vi "Multimetr-facade.vi"(0 "Data In":T4, 2 "Display State In":T2 {"Mode" items=["U DC", "U AC", "I DC", "I AC", "R"]}, 3 "Container State":T3) -> (6 "Data Out":T4, 7 "Display State Out":T2 {"Mode" items=["U DC", "U AC", "I DC", "I AC", "R"]}, 8 "Action":T1)   [LabVIEW 2020, in "Multimetr.xctl"]
uses:
  Multimetr.xctl
  Multimetr-data.ctl
  <vilib>/_xctls/Container State.ctl
  Multimetr-state.ctl
  <vilib>/_xctls/Action.ctl
  <vilib>/_xctls/XControlSupport.lvlib
panel:
  out "U/I/R":dbl
  in  "Power":bool
  in  "Knob":u8(knob)=3 min=3 max=7 step=1 scale=0.0..10.0
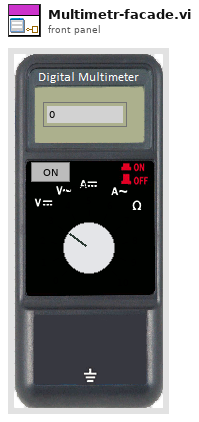
[diagram p1: front panel]
types:
  T1 = typedef "XControlSupport.lvlib/Action.ctl" = cluster{"Data Changed?":bool, "State Changed?":bool, "Action Name":string}
  T2 = typedef "Multimetr.xctl/Multimetr-state.ctl" = cluster{"ON":bool, "Mode":u16, "I connected?":bool, "U connected?":bool}
  T3 = typedef "XControlSupport.lvlib/Container State.ctl" = cluster{"Indicator?":bool, "Run Mode?":bool, " Refnum":refnum<vi>}
  T4 = typedef "Multimetr.xctl/Multimetr-data.ctl" = cluster{"Data":dbl, "Power":bool}
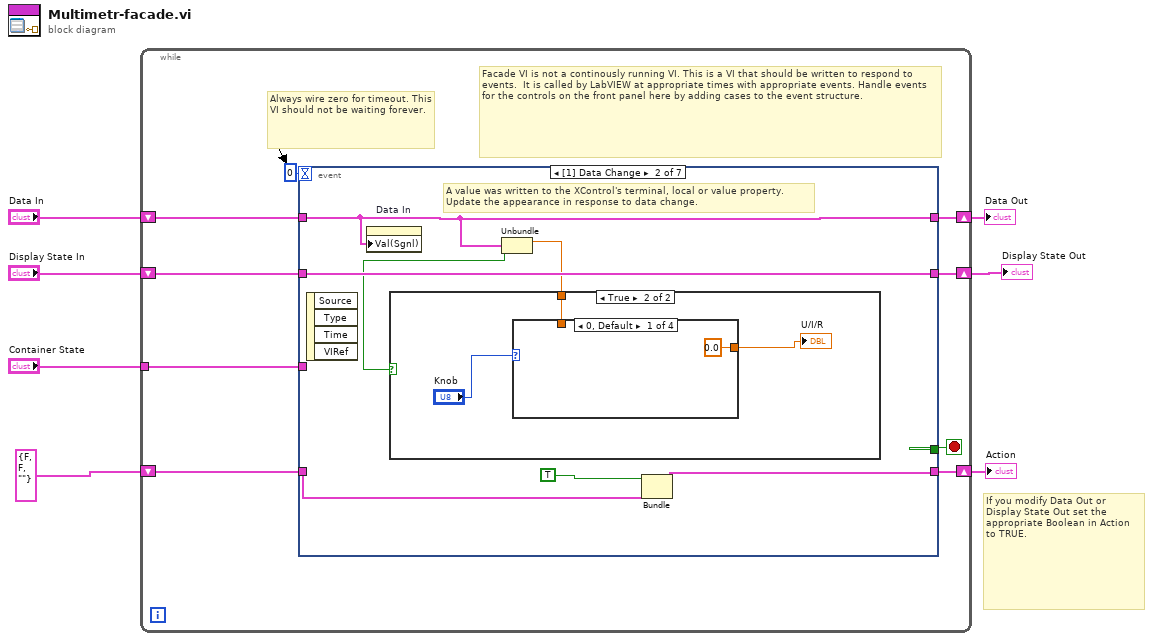
[diagram p0: block diagram]
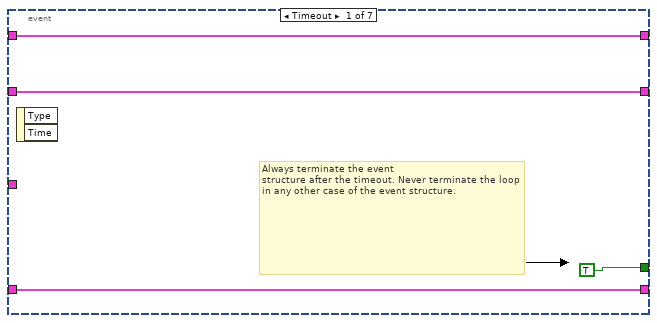
[diagram p2: hidden frame]
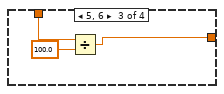
[diagram p5: hidden frame]
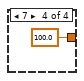
[diagram p6: hidden frame]
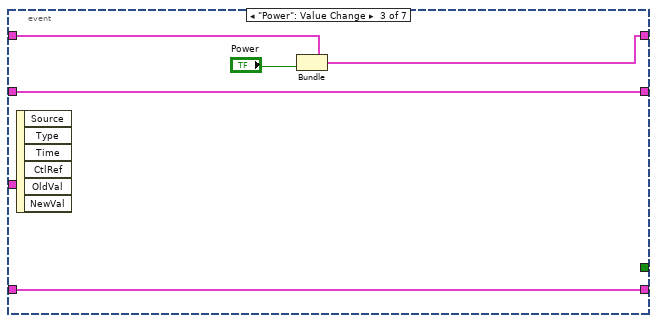
[diagram p7: hidden frame]
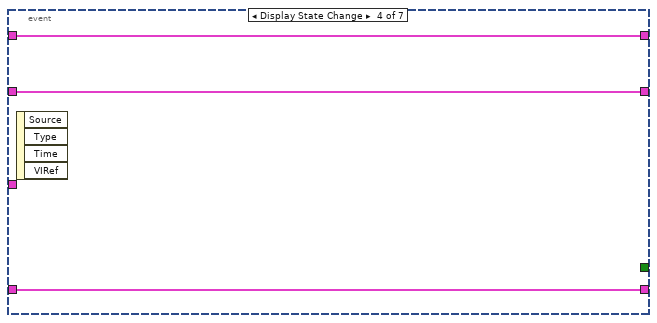
[diagram p8: hidden frame]
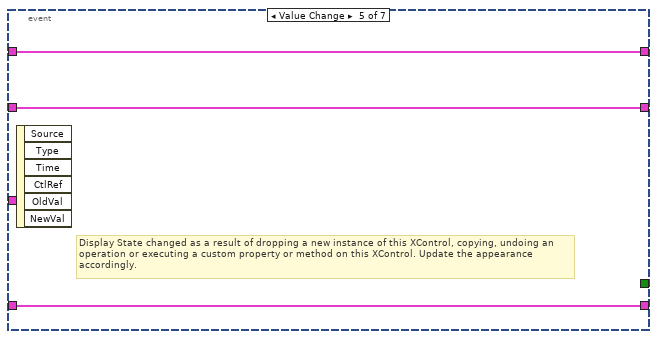
[diagram p9: hidden frame]
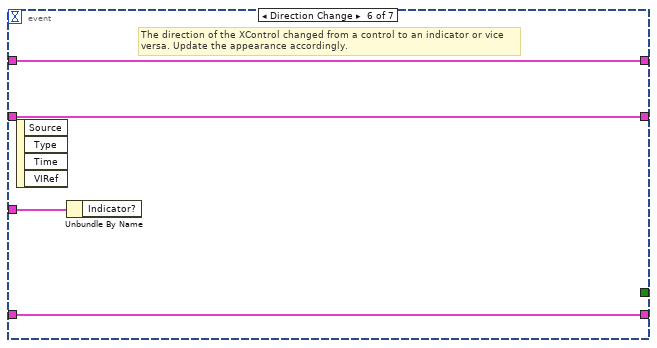
[diagram p10: hidden frame]
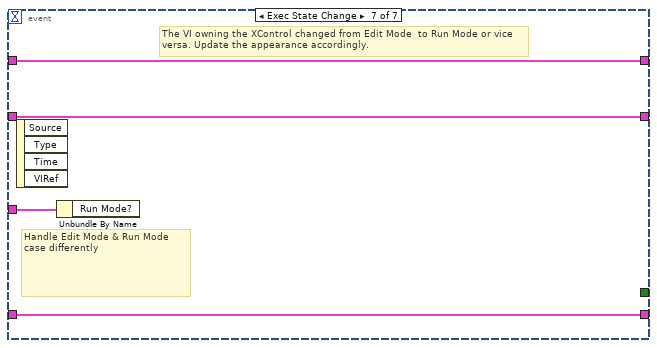
[diagram p11: hidden frame]
diagram:
  # "If you modify Data Out or\nDisplay State Out set the\nappropriate Boolean in Action\nto TRUE."
  n1 = while {
    shift-right: [w15] -> w4
    shift-left: "Display State In" -> [w16]
    tunnel: "Container State" -> [w12]
    shift-right: [w10] -> w7
    shift-left: "Data In" -> [w11]
    shift-right: [w8] -> w2
    shift-left: T1 {"Data Changed?"=FALSE, "State Changed?"=FALSE, "Action Name"=""} ("Action") -> [w9]
    stop <- w14 stop-if-true
    # "Facade VI is not a continously running VI. This is a VI that should be written to respond to events.  It is called by LabVIEW at appropriate times with appropriate events. Handle events for the controls on the front panel here by adding cases to the event structure."
    # "Always wire zero for timeout. This\nVI should not be waiting forever."
    n2 = event shown="[1] Data Change" {
      selector: _ -> [_ _ _ _ _ _ _]
      dyn-events: _ -> [_ _ _ _ _ _ _]
      timeout: 0 -> [_ _ _ _ _ _ _]
      tunnel: w16 -> [w18 w27 w41 w43 w47 w50 w54]
      tunnel: [w18 w27 w41 w43 w47 w50 w54] -> w15
      tunnel: [TRUE _ _ _ _ _ _] -> w14
      tunnel: w12 -> [_ _ _ _ _ w51 w55]
      tunnel: w11 -> [w17 w21 w39 w44 w46 w49 w53]
      tunnel: [w17 w21 w37 w44 w46 w49 w53] -> w10
      tunnel: [w19 w25 w40 w42 w45 w48 w52] -> w8
      tunnel: w9 -> [w19 w26 w40 w42 w45 w48 w52]
      event Timeout {
        # "Always terminate the event\nstructure after the timeout. Never terminate the loop in any other case of the event structure."
        n3 = event-data() -> ()  [unwired: 1 in, 2 out]
      }
      event Data Change {
        # "A value was written to the XControl's terminal, local or value property.\nUpdate the appearance in response to data change."
        n4 = event-data() -> ()  [unwired: 1 in, 4 out]
        n5 = property on="Data In" class="Clust (strict)"("Val(Sgnl)"=w21) -> ()  [unwired: 2 in, 2 out]
        n6 = Unbundle(w21) -> ("Data"=w23:dbl, "Power"=w22:bool)
        n7 = case shown="True" w22 {
          tunnel: w23 -> [_ w30]
          frame False {
          }
          frame True {
            n8 = case shown="0, Default" "Knob" {
              tunnel: [0.0 ("U/I/R") w32 w33 100.0 ("U/I/R")] -> w28
              tunnel: w30 -> [_ w32 w35 _]
              frame 0, Default {
              }
              frame 3, 4 {
              }
              frame 5, 6 {
                n9 = Divide(x=w35, y=100.0) -> (x/y=w33:dbl)
              }
              frame 7 {
              }
            }
            "U/I/R" <- w28
          }
        }
        n10 = Bundle(cluster=w26, "Data Changed?"=TRUE) -> (w25:T1)  [unwired: 2 in]
      }
      event "Power": Value Change {
        n11 = event-data() -> ()  [unwired: 1 in, 6 out]
        n12 = Bundle(cluster=w39, "Power"="Power") -> (w37:T4)  [unwired: 1 in]
      }
      event Display State Change {
        n13 = event-data() -> ()  [unwired: 1 in, 4 out]
      }
      event Value Change {
        # "Display State changed as a result of dropping a new instance of this XControl, copying, undoing an operation or executing a custom property or method on this XControl. Update the appearance accordingly."
        n14 = event-data() -> ()  [unwired: 1 in, 6 out]
      }
      event Direction Change {
        # "The direction of the XControl changed from a control to an indicator or vice versa. Update the appearance accordingly."
        n15 = event-data() -> ()  [unwired: 1 in, 4 out]
        n16 = Unbundle By Name(w51) -> ()  [unwired: 1 out]
      }
      event Exec State Change {
        # "The VI owning the XControl changed from Edit Mode  to Run Mode or vice versa. Update the appearance accordingly."
        # "Handle Edit Mode & Run Mode\ncase differently"
        n17 = event-data() -> ()  [unwired: 1 in, 4 out]
        n18 = Unbundle By Name(w55) -> ()  [unwired: 1 out]
      }
    }
  }
  "Display State Out" <- w4
  "Data Out" <- w7
  "Action" <- w2
